vi "get Analog Config Ver3.vi"(7 "analogIndex":i32, 9 "pmuIndex":i32, 10 "pseudoPdcId":i32, 11 "analogCfg":T1) -> (1 "function return":i32, 2 "name":string, 3 "analogCfg out":T1)   [LabVIEW 2013, in "C37118-DLL.lvlib" / "StrongridDLL.lvlib"]
doc: "STRONGRIDIEEEC37118DLL_API int __cdecl getAnalogConfig_Ver3(analogConfig_Ver3 *analogCfg, int32_t pseudoPdcId, int32_t pmuIndex, int32_t analogIndex);"
uses:
  StrongridDLL.lvlib
  StrongridDLL/StrongridDLL.dll
  <vilib>/Utility/importsl/GetValueByPointer/GetValueByPointer.xnode
  <vilib>/Utility/importsl/GetValueByPointer/datatype.ctl
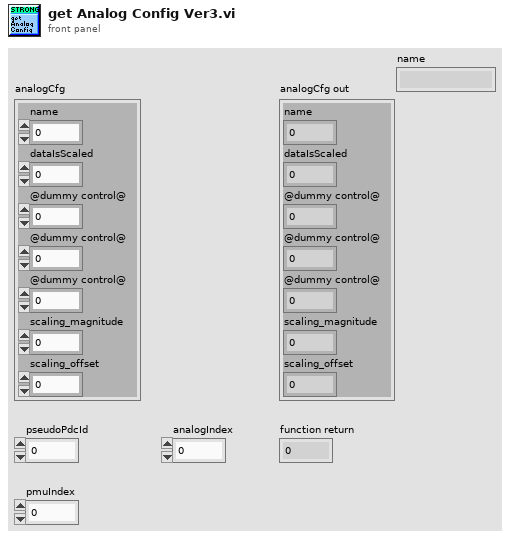
[diagram p1: front panel]
types:
  T1 = cluster{"name":u32, "dataIsScaled":u8, "@dummy control@":i8, "@dummy control@":i8, "@dummy control@":i8, "scaling_magnitude":sgl, "scaling_offset":sgl}
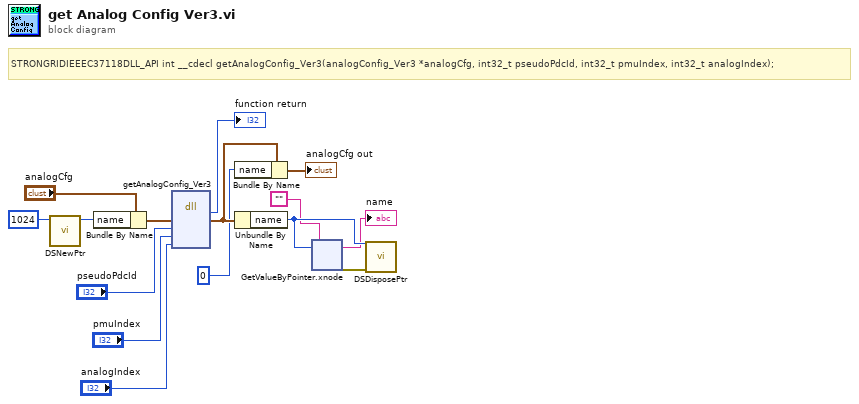
[diagram p0: block diagram]
diagram:
  # "STRONGRIDIEEEC37118DLL_API int __cdecl getAnalogConfig_Ver3(analogConfig_Ver3 *analogCfg, int32_t pseudoPdcId, int32_t pmuIndex, int32_t analogIndex);"
  n1 = call <vilib>:"DSNewPtr.vi"("Size"=u64 1024) -> ("Pointer"=w12:u64)  [unwired: 9 in, 1 out]
  n2 = Bundle By Name(cluster="analogCfg", "name"=w12) -> (w11:T1)
  n3 = dll-call lib="C:/dev/OSS/S3DK/builds/StrongridDLL/StrongridDLL.*" fn="getAnalogConfig_Ver3"("analogCfg"=w11, "pseudoPdcId"="pseudoPdcId", "pmuIndex"="pmuIndex", "analogIndex"="analogIndex") -> (→"function return":i32, "analogCfg"=w6:T1)  [unwired: 6 in, 2 out]
  n4 = Bundle By Name(cluster=w6, "name"=u32 0) -> (→"analogCfg out":T1)
  n5 = Unbundle By Name(w6) -> ("name"=w9:u32)
  n6 = xnode "GetValueByPointer.xnode"("Pointer"=w9, "InputType"="") -> ("Output"=→"name":string, "ErrorOut"=w10:errorcluster)  [unwired: 2 in]
  n7 = call <vilib>:"DSDisposePtr.vi"("error in (no error)"=w10, "Pointer"=w9) -> ()  [unwired: 9 in, 1 out]
